vi "Cambridge Laser Control.vi"(7 "Calling VI Ref":refnum<vi>) -> ()   [LabVIEW 2016]
uses:
  Laser Controls/Laser Control.ctl
  Laser Controls/AOTF Control.ctl
  <vilib>/Utility/miscctls.llb/LVPointTypeDef.ctl
  Hardware Configuration/Hardware Configuration Controls/Device Type.ctl
  Hardware Configuration/Hardware Configuration Controls/Device Function.ctl
  Device Library/Lasers/Laser Controls/Laser Actions.ctl
  Device Library/AOTF and AOM/AOTF Controls/AOTF Actions.ctl
panel:
  in  "642 AOTF":T1 {"Power (%)" max=100 step=1 scale=0.0..100.0; "Digital Power (%)" max=100 step=1}
  in  "560 AOTF":T1 {"Power (%)" max=100 step=1 scale=0.0..100.0; "Digital Power (%)" max=100 step=1}
  in  "546 AOTF":T1 {"Power (%)" max=100 step=1 scale=0.0..100.0; "Digital Power (%)" max=100 step=1}
  in  "488 AOTF":T1 {"Power (%)" max=100 step=1 scale=0.0..100.0; "Digital Power (%)" max=100 step=1}
  in  "405 AOTF":T1 {"Power (%)" max=100 step=1 scale=0.0..100.0; "Digital Power (%)" max=100 step=1}
  in  "Lasers On/Off":bool
  in  "Quit":bool
  in  "642":T2
  in  "560":T2
  in  "546":T2
  in  "488":T2
  in  "405":T2
  # "Laser Status"
  # "Laser Emission"
  # "Laser Power"
  # "Capture Active"
  # "Power (%)"
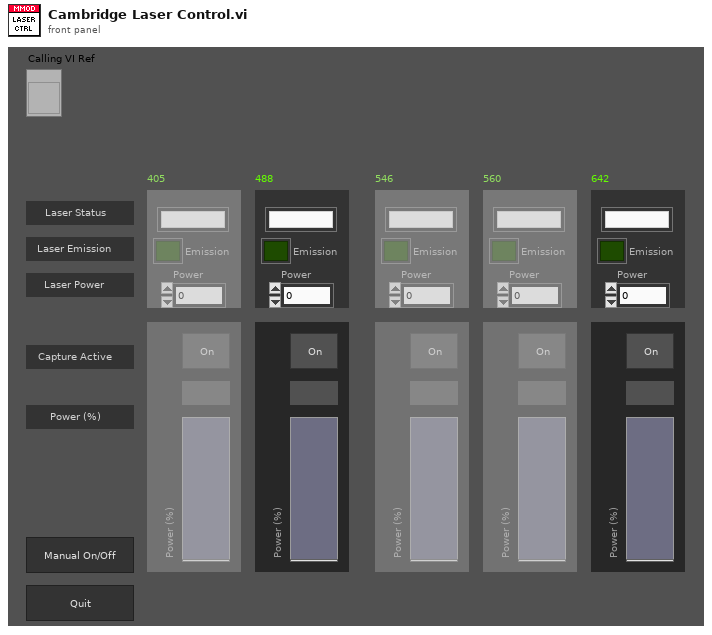
[diagram p1: front panel]
types:
  T1 = typedef "AOTF Control.ctl" = cluster{"Active":bool, "Digital Power (%)":u8, "Power (%)":u8}
  T2 = typedef "Laser Control.ctl" = cluster{"Status":string, "Emission":bool, "Power":dbl}
  T3 = enum16{"Always On", "Always Off", "Off While Running"}
  T4 = typedef "LVPointTypeDef.ctl" = cluster{"Horizontal":i16, "Vertical":i16}
  T5 = typedef "Device Function.ctl" = enum16{"Primary", "Secondary", "Overview", "Wide Field Drift Correction", "642 nm Excitation", "560 nm Excitation", "546 nm Excitation", "488 nm Excitation", "405 nm Excitation", "Objective Drift Correction", "Objective XY", "Objective Z", "Sample XY", "Sample Coarse Z", "Sample Z", "4Pi Lower", "4Pi Upper", "Adj Cavity"}
  T6 = typedef "Device Type.ctl" = enum16{"AOTF", "Camera", "Deformable Mirror", "Laser", "Shutter", "Stage"}
  T7 = typedef "Laser Actions.ctl" = enum16{"Error Check", "Set On/Off", "Set Power", "Set Parameter", "Get Power", "Get Status", "Get Parameter", "Quit"}
  T8 = enum8{"Enabled", "Disabled", "Disabled and Grayed Out"}
  T9 = typedef "AOTF Actions.ctl" = enum16{"Error Check", "Blank", "Line On/Off", "Set Power", "Status", "Quit"}
  T10 = typedef "Laser Status.ctl" = enum16{"Warmup", "Ready", "Emission", "Tuning", "Error"}
  T11 = cluster{"Status":bool, "Emission":bool, "Power":bool}
  T12 = cluster{"Active":bool, "Digital Power (%)":bool, "Power (%)":bool}
  T13 = typedef "LVRectTypeDef.ctl" = cluster{"Left":i16, "Top":i16, "Right":i16, "Bottom":i16}
  T14 = typedef "LVBoundsTypeDef.ctl" = cluster{"Width":u32, "Height":u32}
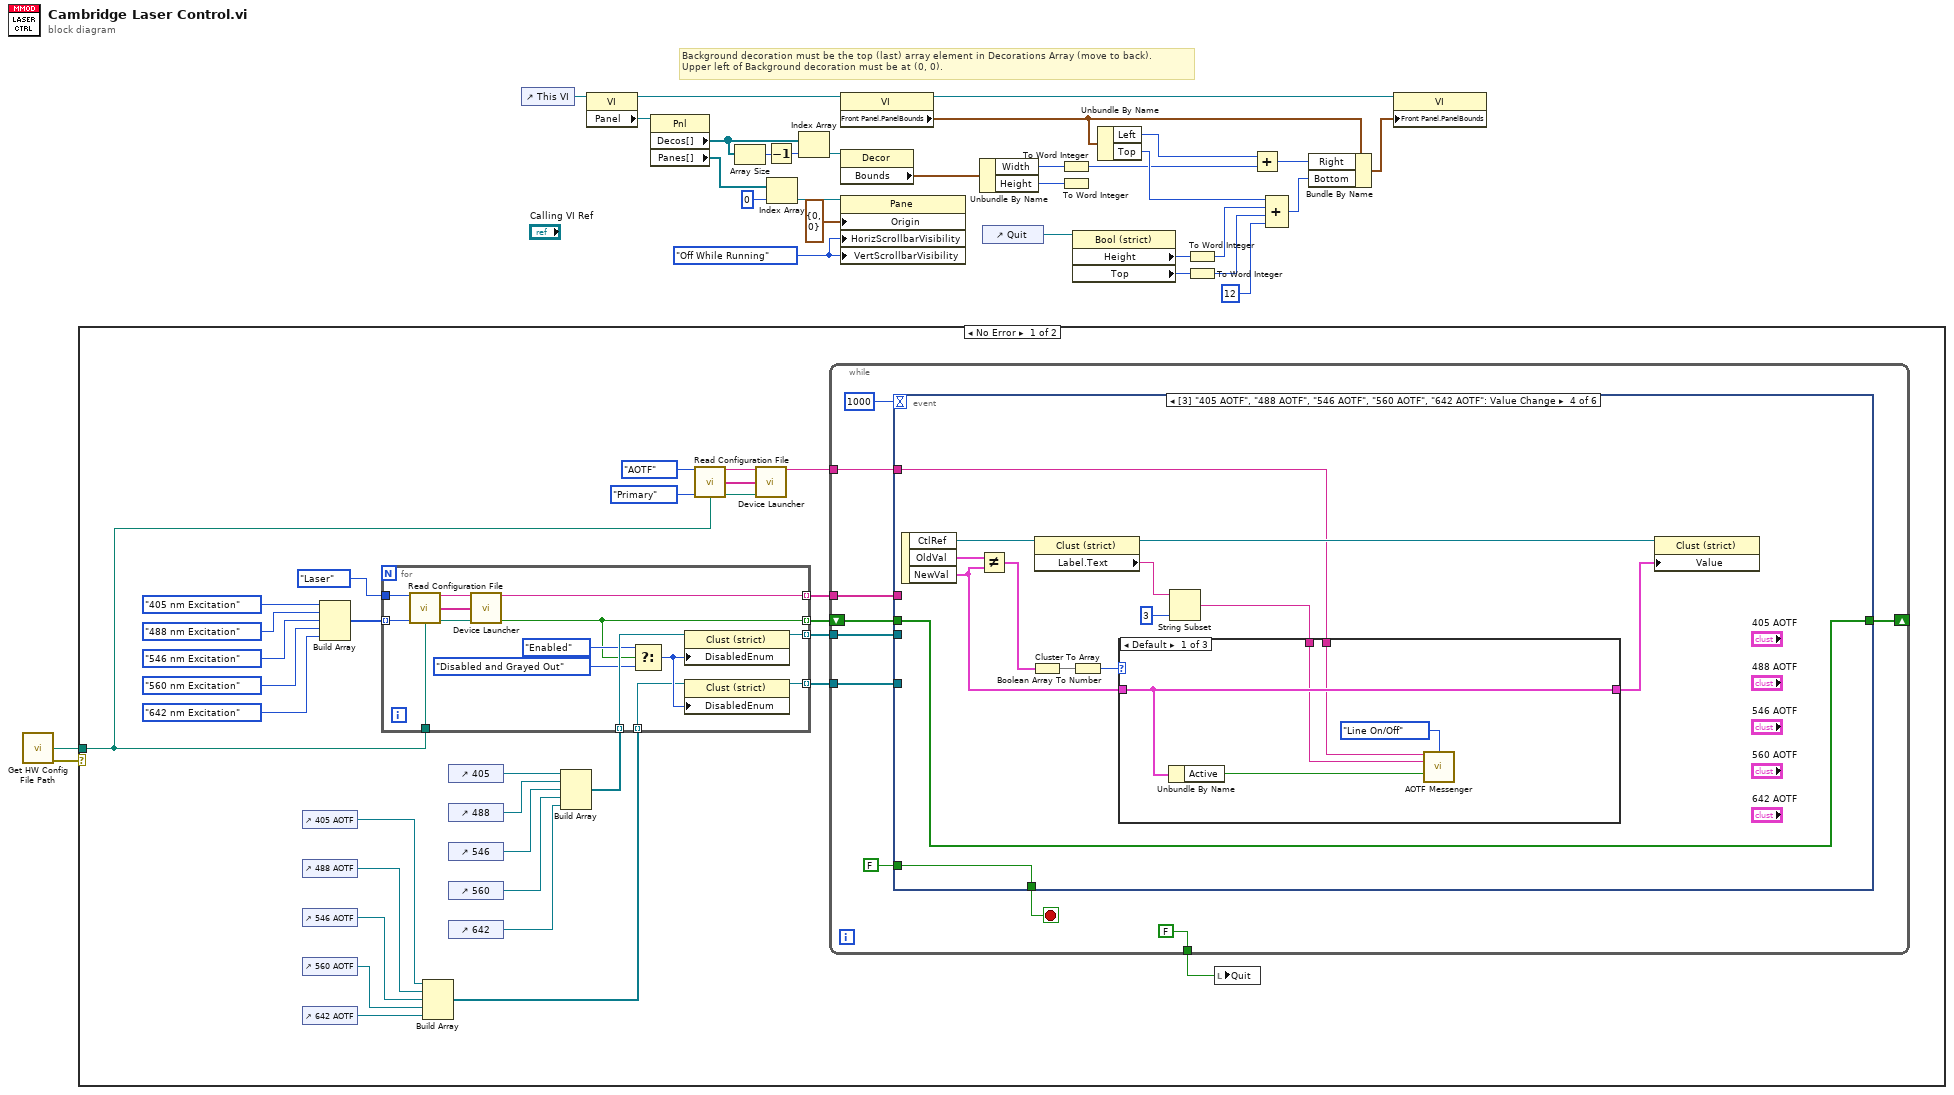
[diagram p0: block diagram]
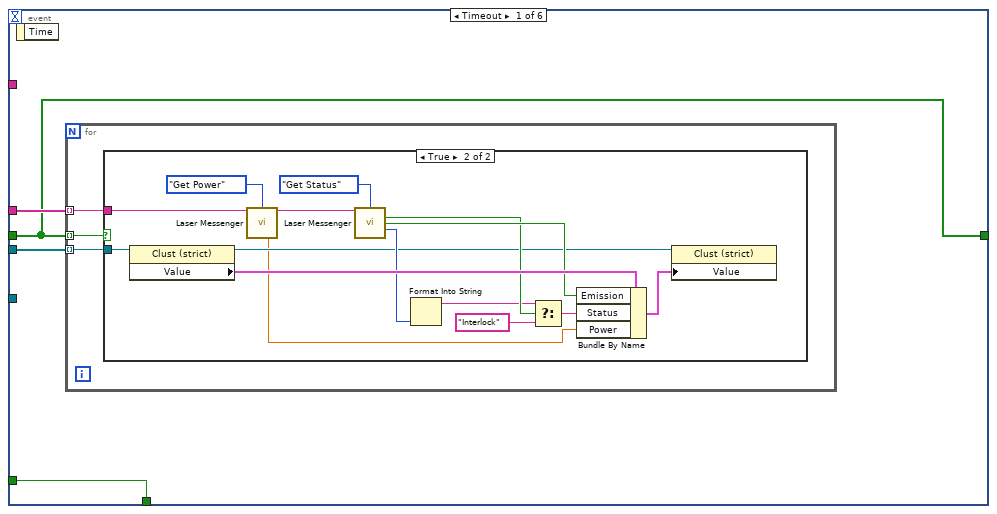
[diagram p2: hidden frame]
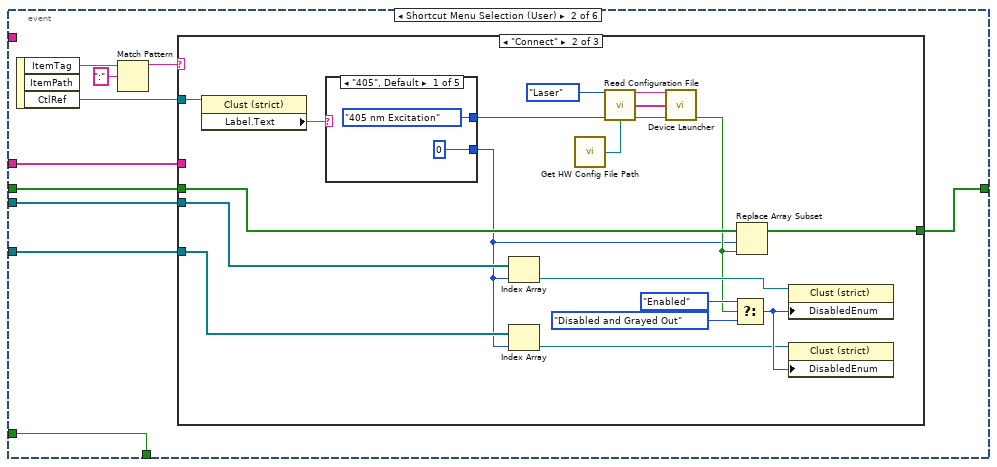
[diagram p4: hidden frame]
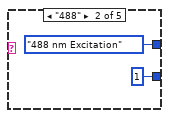
[diagram p6: hidden frame]
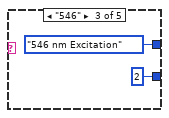
[diagram p7: hidden frame]
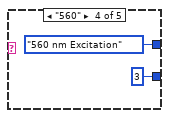
[diagram p8: hidden frame]
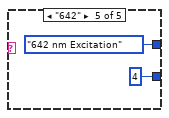
[diagram p9: hidden frame]
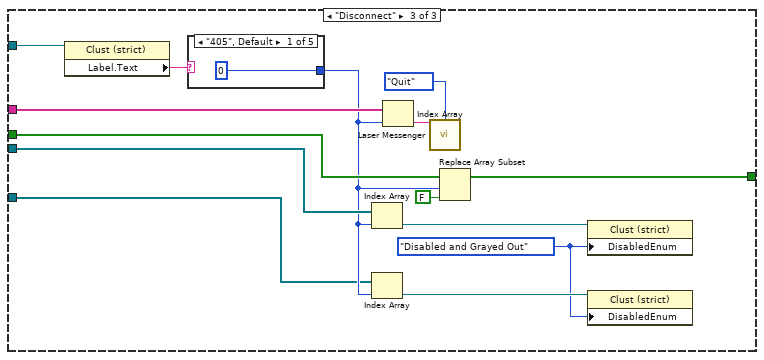
[diagram p10: hidden frame]
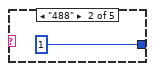
[diagram p11: hidden frame]
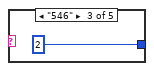
[diagram p12: hidden frame]
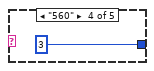
[diagram p13: hidden frame]
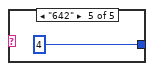
[diagram p14: hidden frame]
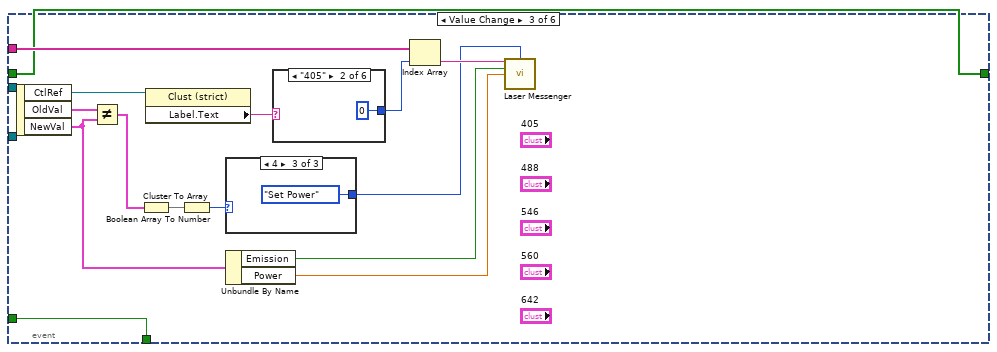
[diagram p15: hidden frame]
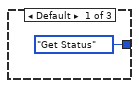
[diagram p16: hidden frame]
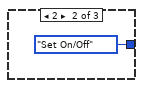
[diagram p17: hidden frame]
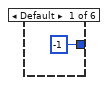
[diagram p18: hidden frame]
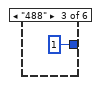
[diagram p19: hidden frame]
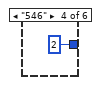
[diagram p20: hidden frame]
diagram:
  w12 = T3."Off While Running" ("Vertical Scrollbar Visibility")
  # "Background decoration must be the top (last) array element in Decorations Array (move to back).\nUpper left of Background decoration must be at (0, 0)."
  n1 = call "Get HW Config File Path.vi"() -> ("File Path"=w30:path, "Error"=w31:errorcluster)  [unwired: 14 in]
  n2 = case shown="No Error" w31 {
    tunnel: w30 -> [w32 _]
    frame No Error {
      n3 = control-ref of="405 AOTF"() -> (w42:refnum<vi>)
      n4 = control-ref of="488 AOTF"() -> (w43:refnum<vi>)
      n5 = control-ref of="546 AOTF"() -> (w44:refnum<vi>)
      n6 = control-ref of="560 AOTF"() -> (w45:refnum<vi>)
      n7 = control-ref of="642 AOTF"() -> (w46:refnum<vi>)
      n8 = Build Array(Device_Function."405 nm Excitation" ("Device Function"), Device_Function."488 nm Excitation" ("Device Function"), Device_Function."546 nm Excitation" ("Device Function"), Device_Function."560 nm Excitation" ("Device Function"), Device_Function."642 nm Excitation" ("Device Function")) -> (w56:T5[])
      n9 = Build Array(w42, w43, w44, w45, w46) -> (w41:refnum<vi>[])
      n10 = control-ref of="405"() -> (w51:refnum<vi>)
      n11 = control-ref of="488"() -> (w55:refnum<vi>)
      n12 = control-ref of="546"() -> (w54:refnum<vi>)
      n13 = control-ref of="560"() -> (w53:refnum<vi>)
      n14 = control-ref of="642"() -> (w52:refnum<vi>)
      n15 = Build Array(w51, w55, w54, w53, w52) -> (w50:refnum<vi>[])
      n16 = for {
        tunnel: [w236] -> w49 mode=indexing
        tunnel: Device_Type."Laser" ("Device Type") -> [w235]
        tunnel: w56 -> [w234] mode=indexing
        tunnel: w32 -> [w233]
        tunnel: w50 -> [w232] mode=indexing
        tunnel: [w229] -> w48 mode=indexing
        tunnel: [w228] -> w47 mode=indexing
        tunnel: w41 -> [w226] mode=indexing
        tunnel: [w225] -> w33 mode=indexing
        n17 = call "Read Configuration File.vi"("Device Type"=w235, "Device Function"=w234, "Config File Path"=w233) -> ("Unique Notifier Name"=w239:string, "Device Ports/IDs/Channels"=w237:string[], "Device Engine Path"=w238:path)  [unwired: 9 in, 1 out]
        n18 = call "Device Launcher.vi"("Notifier Name"=w239, "Device Ports/IDs/Channels"=w237, "Device Engine Path"=w238) -> ("Notifier Name"=w236:string, "Running?"=w229:bool)  [unwired: 11 in]
        n19 = Select(t=T8."Enabled" ("Disabled"), s=w229, f=T8."Disabled and Grayed Out") -> (s? t:f=w227:T8)
        n20 = property class="Clust (strict)"(reference=w232, "DisabledEnum"=w227) -> (reference out=w228:refnum<vi>)  [unwired: 1 in, 1 out]
        n21 = property class="Clust (strict)"(reference=w226, "DisabledEnum"=w227) -> (reference out=w225:refnum<vi>)  [unwired: 1 in, 1 out]
      }
      n22 = call "Read Configuration File.vi"("Device Type"=Device_Type."AOTF", "Device Function"=Device_Function."Primary", "Config File Path"=w32) -> ("Unique Notifier Name"=w38:string, "Device Ports/IDs/Channels"=w40:string[], "Device Engine Path"=w39:path)  [unwired: 9 in, 1 out]
      n23 = call "Device Launcher.vi"("Notifier Name"=w38, "Device Ports/IDs/Channels"=w40, "Device Engine Path"=w39) -> ("Notifier Name"=w35:string)  [unwired: 11 in, 1 out]
      n24 = while {
        tunnel: w49 -> [w71]
        tunnel: w47 -> [w67]
        shift-right: [w66] -> _
        shift-left: w48 -> [w70]
        tunnel: w35 -> [w65]
        tunnel: [FALSE] -> w34
        tunnel: w33 -> [w63]
        stop <- w68 stop-if-true
        n25 = event shown="[3] \"405 AOTF\", \"488 AOTF\", \"546 AOTF\", \"560 AOTF\", \"642 AOTF\": Value Change" {
          selector: _ -> [_ _ _ _ _ _]
          dyn-events: _ -> [_ _ _ _ _ _]
          timeout: 1000 -> [_ _ _ _ _ _]
          tunnel: w71 -> [w75 w96 w165 _ _ w218]
          tunnel: w70 -> [w73 w100 w154 w180 w212 w217]
          tunnel: FALSE -> [w76 w98 w168 w191 w215 _]
          tunnel: [w76 w98 w168 w191 w215 w219] -> w68
          tunnel: w67 -> [w74 w97 _ _ _ _]
          tunnel: [w73 w99 w154 w180 w212 w216] -> w66
          tunnel: w65 -> [_ _ _ w178 w214 _]
          tunnel: w63 -> [_ w95 _ _ _ _]
          event Timeout {
            n26 = event-data() -> ()  [unwired: 1 in, 1 out]
            n27 = for {
              tunnel: w75 -> [w78] mode=indexing
              tunnel: w73 -> [w79] mode=indexing
              tunnel: w74 -> [w77] mode=indexing
              n28 = case shown="True" w79 {
                tunnel: w78 -> [_ w84]
                tunnel: w77 -> [_ w93]
                frame False {
                }
                frame True {
                  n29 = property class="Clust (strict)"(reference=w93) -> (reference out=w85:refnum<vi>, "Value"=w92:T2)  [unwired: 1 in, 1 out]
                  n30 = call "Laser Messenger.vi"("Notifier Name"=w84, "Action"=Laser_Actions."Get Power") -> ("Notifier Name Dup"=w83:string, "Power (mW)"=w81:dbl)  [unwired: 8 in, 4 out]
                  n31 = call "Laser Messenger.vi"("Notifier Name"=w83, "Action"=Laser_Actions."Get Status") -> ("Enabled (Interlock)?"=w89:bool, "Light Emission?"=w91:bool, "Laser Status"=w90:T10)  [unwired: 8 in, 3 out]
                  n32 = Format Into String(w90) -> (resulting string=w88:string)  [unwired: 3 in, 1 out]
                  n33 = Select(t=w88, s=w89, f="Interlock") -> (s? t:f=w86:string)
                  n34 = Bundle By Name(cluster=w92, "Emission"=w91, "Status"=w86, "Power"=w81) -> (w80:T2)
                  n35 = property class="Clust (strict)"(reference=w85, "Value"=w80) -> ()  [unwired: 1 in, 2 out]
                }
              }
            }
          }
          event Shortcut Menu Selection (User) {
            n36 = event-data() -> ("ItemTag"=w103:string, "CtlRef"=w101:refnum<vi>)  [unwired: 1 in, 1 out]
            n37 = Match Pattern(string=w103, regular expression=":") -> (before substring=w102:string)  [unwired: 1 in, 3 out]
            n38 = case shown="\"Connect\"" w102 {
              tunnel: w101 -> [_ w124 w145]
              tunnel: w100 -> [w105 w117 w144]
              tunnel: [w105 w113 w142] -> w99
              tunnel: w97 -> [_ w112 w146]
              tunnel: w96 -> [_ _ w143]
              tunnel: w95 -> [_ w108 w137]
              frame Default {
              }
              frame "Connect" {
                n39 = property class="Clust (strict)"(reference=w124) -> ("Label.Text"=w123:string)  [unwired: 1 in, 2 out]
                n40 = case shown="\"405\", Default" w123 {
                  tunnel: [Device_Function."405 nm Excitation" ("Device Function") Device_Function."488 nm Excitation" ("Device Function") Device_Function."546 nm Excitation" ("Device Function") Device_Function."560 nm Excitation" ("Device Function") Device_Function."642 nm Excitation" ("Device Function")] -> w119
                  tunnel: [0 1 2 3 4] -> w107
                  frame "405", Default {
                  }
                  frame "488" {
                  }
                  frame "546" {
                  }
                  frame "560" {
                  }
                  frame "642" {
                  }
                }
                n41 = Index Array(array=w112, index=w107) -> (element=w111:refnum<vi>)
                n42 = Index Array(array=w108, index=w107) -> (element=w106:refnum<vi>)
                n43 = call "Get HW Config File Path.vi"() -> ("File Path"=w118:path)  [unwired: 14 in, 1 out]
                n44 = call "Read Configuration File.vi"("Device Type"=Device_Type."Laser", "Device Function"=w119, "Config File Path"=w118) -> ("Unique Notifier Name"=w120:string, "Device Ports/IDs/Channels"=w122:string[], "Device Engine Path"=w121:path)  [unwired: 9 in, 1 out]
                n45 = call "Device Launcher.vi"("Notifier Name"=w120, "Device Ports/IDs/Channels"=w122, "Device Engine Path"=w121) -> ("Running?"=w110:bool)  [unwired: 11 in, 1 out]
                n46 = Select(t=T8."Enabled" ("Disabled"), s=w110, f=T8."Disabled and Grayed Out") -> (s? t:f=w109:T8)
                n47 = Replace Array Subset(array=w117, new element=w110, index=w107) -> (w113:bool[])
                n48 = property class="Clust (strict)"(reference=w111, "DisabledEnum"=w109) -> ()  [unwired: 1 in, 2 out]
                n49 = property class="Clust (strict)"(reference=w106, "DisabledEnum"=w109) -> ()  [unwired: 1 in, 2 out]
              }
              frame "Disconnect" {
                w135 = T8."Disabled and Grayed Out" ("Disabled")
                n50 = property class="Clust (strict)"(reference=w145) -> ("Label.Text"=w148:string)  [unwired: 1 in, 2 out]
                n51 = case shown="\"405\", Default" w148 {
                  tunnel: [0 1 2 3 4] -> w138
                  frame "405", Default {
                  }
                  frame "488" {
                  }
                  frame "546" {
                  }
                  frame "560" {
                  }
                  frame "642" {
                  }
                }
                n52 = Index Array(array=w146, index=w138) -> (element=w147:refnum<vi>)
                n53 = Index Array(array=w137, index=w138) -> (element=w136:refnum<vi>)
                n54 = Index Array(array=w143, index=w138) -> (element=w141:string)
                n55 = call "Laser Messenger.vi"("Notifier Name"=w141, "Action"=Laser_Actions."Quit") -> ()  [unwired: 8 in, 6 out]
                n56 = Replace Array Subset(array=w144, new element=FALSE ("new element/subarray"), index=w138) -> (w142:bool[])
                n57 = property class="Clust (strict)"(reference=w147, "DisabledEnum"=w135) -> ()  [unwired: 1 in, 2 out]
                n58 = property class="Clust (strict)"(reference=w136, "DisabledEnum"=w135) -> ()  [unwired: 1 in, 2 out]
              }
            }
          }
          event Value Change {
            n59 = event-data() -> ("CtlRef"=w167:refnum<vi>, "OldVal"=w163:T2, "NewVal"=w157:T2)  [unwired: 1 in]
            n60 = Not Equal?(x=w163, y=w157) -> (x != y?=w158:T11)
            n61 = Cluster To Array(cluster=w158) -> (array=w162:bool[])
            n62 = property class="Clust (strict)"(reference=w167) -> ("Label.Text"=w166:string)  [unwired: 1 in, 2 out]
            n63 = Boolean Array To Number(Boolean array=w162) -> (number=w161:u32)
            n64 = case shown="4" w161 {
              tunnel: [Laser_Actions."Get Status" ("Action") Laser_Actions."Set On/Off" ("Action") Laser_Actions."Set Power" ("Action")] -> w159
              frame Default {
              }
              frame 2 {
              }
              frame 4 {
              }
            }
            n65 = Unbundle By Name(w157) -> ("Emission"=w155:bool, "Power"=w156:dbl)
            n66 = case shown="\"405\"" w166 {
              tunnel: [-1 0 1 2 3 4] -> w164
              frame Default {
              }
              frame "405" {
              }
              frame "488" {
              }
              frame "546" {
              }
              frame "560" {
              }
              frame "642" {
              }
            }
            n67 = Index Array(array=w165, index=w164) -> (element=w160:string)
            n68 = call "Laser Messenger.vi"("Notifier Name"=w160, "Action"=w159, "Emission On/Off"=w155, "Power (mW)"=w156) -> ()  [unwired: 6 in, 6 out]
          }
          event Value Change {
            n69 = event-data() -> ("CtlRef"=w188:refnum<vi>, "OldVal"=w187:T1, "NewVal"=w183:T1)  [unwired: 1 in]
            n70 = Not Equal?(x=w187, y=w183) -> (x != y?=w189:T12)
            n71 = Cluster To Array(cluster=w189) -> (array=w190:bool[])
            n72 = property class="Clust (strict)"(reference=w188) -> (reference out=w182:refnum<vi>, "Label.Text"=w186:string)  [unwired: 1 in, 1 out]
            n73 = Boolean Array To Number(Boolean array=w190) -> (number=w184:u32)
            n74 = String Subset(string=w186, length (rest)=3 ("length (rest)")) -> (substring=w179:string)  [unwired: 1 in]
            n75 = case shown="Default" w184 {
              tunnel: w183 -> [w196 w202 w210]
              tunnel: [w196 w203 w209] -> w181
              tunnel: w179 -> [w192 w200 w206]
              tunnel: w178 -> [w193 w199 w207]
              frame Default {
                n76 = Unbundle By Name(w196) -> ("Active"=w194:bool)
                n77 = call "AOTF Messenger.vi"("AOTF Notifier Name"=w193, "AOTF Action"=AOTF_Actions."Line On/Off", "Wavelength (nm)"=w192, "Line On/Off"=w194) -> ()  [unwired: 7 in, 5 out]
              }
              frame 2 {
                n78 = Unbundle By Name(w202) -> ("Digital Power (%)"=w198:u8)
                n79 = To Double Precision Float(number=w198) -> (double precision float=w197:dbl)
                n80 = Bundle By Name(cluster=w202, "Power (%)"=w198) -> (w203:T1)
                n81 = call "AOTF Messenger.vi"("AOTF Notifier Name"=w199, "AOTF Action"=AOTF_Actions."Set Power", "Wavelength (nm)"=w200, "Power (%)"=w197) -> ()  [unwired: 7 in, 5 out]
              }
              frame 4 {
                n82 = Unbundle By Name(w210) -> ("Power (%)"=w205:u8)
                n83 = To Double Precision Float(number=w205) -> (double precision float=w204:dbl)
                n84 = Bundle By Name(cluster=w210, "Digital Power (%)"=w205) -> (w209:T1)
                n85 = call "AOTF Messenger.vi"("AOTF Notifier Name"=w207, "AOTF Action"=AOTF_Actions."Set Power", "Wavelength (nm)"=w206, "Power (%)"=w204) -> ()  [unwired: 7 in, 5 out]
              }
            }
            n86 = property class="Clust (strict)"(reference=w182, "Value"=w181) -> ()  [unwired: 1 in, 2 out]
          }
          event "Lasers On/Off": Value Change {
            n87 = event-data() -> ()  [unwired: 1 in, 6 out]
            n88 = call "AOTF Messenger.vi"("AOTF Notifier Name"=w214, "AOTF Action"=AOTF_Actions."Blank", "Beam Blank"="Lasers On/Off") -> ()  [unwired: 8 in, 5 out]
          }
          event "Quit": Value Change {
            n89 = event-data() -> ("NewVal"=w219:bool)  [unwired: 1 in]
            n90 = for {
              tunnel: w218 -> [w221] mode=indexing
              tunnel: w217 -> [w220] mode=indexing
              tunnel: [w220] -> w216 mode=indexing
              n91 = case shown="True" w220 {
                tunnel: w221 -> [_ w224]
                frame False {
                }
                frame True {
                  n92 = call "Laser Messenger.vi"("Notifier Name"=w224, "Action"=Laser_Actions."Set On/Off", "Emission On/Off"=FALSE) -> ()  [unwired: 7 in, 6 out]
                }
              }
            }
          }
        }
      }
      n93 = local write "Quit"(w34) -> ()
    }
    frame Error {
    }
  }
  n94 = control-ref of="This VI"() -> (w4:refnum<vi>)
  n95 = property class="VI"(reference=w4) -> (reference out=w13:refnum<vi>, "Panel"=w5:refnum<vi>)  [unwired: 1 in, 1 out]
  n96 = property class="Pnl"(reference=w5) -> ("Decos[]"=w3:refnum<vi>[], "Panes[]"=w9:refnum<vi>[])  [unwired: 1 in, 2 out]
  n97 = Array Size(array=w3) -> (size(s)=w1:i32)
  n98 = Decrement(x=w1) -> (x-1=w2:i32)
  n99 = Index Array(array=w9, index=0) -> (element=w8:refnum<vi>)
  n100 = Index Array(array=w3, index=w2) -> (element=w11:refnum<vi>)
  n101 = property class="VI"(reference=w13) -> (reference out=w15:refnum<vi>, "Front Panel.PanelBounds"=w16:T13)  [unwired: 1 in, 1 out]
  n102 = property class="Decor"(reference=w11) -> ("Bounds"=w14:T14)  [unwired: 1 in, 2 out]
  n103 = property class="Pane"(reference=w8, "Origin"=T4 {"Horizontal"=0, "Vertical"=0}, "HorizScrollbarVisibility"=w12, "VertScrollbarVisibility"=w12) -> ()  [unwired: 1 in, 2 out]
  n104 = Unbundle By Name(w14) -> ("Width"=w19:u32, "Height"=w22:u32)
  n105 = control-ref of="Quit"() -> (w6:refnum<vi>)
  n106 = To Word Integer(number=w19) -> (16bit integer=w21:i16)
  n107 = To Word Integer(number=w22) -> ()  [unwired: 1 out]
  n108 = property class="Bool (strict)"(reference=w6) -> ("Height"=w24:u32, "Top"=w25:i32)  [unwired: 1 in, 2 out]
  n109 = Unbundle By Name(w16) -> ("Left"=w18:i16, "Top"=w29:i16)
  n110 = To Word Integer(number=w24) -> (16bit integer=w27:i16)
  n111 = To Word Integer(number=w25) -> (16bit integer=w28:i16)
  n112 = Add(x=w18, y=w21) -> (x+y=w20:i16)
  n113 = Compound Arithmetic op=ADD(w29, w27, w28, i16 12 ("y")) -> (w23:i16)
  n114 = Bundle By Name(cluster=w16, "Right"=w20, "Bottom"=w23) -> (w17:T13)
  n115 = property class="VI"(reference=w15, "Front Panel.PanelBounds"=w17) -> ()  [unwired: 1 in, 2 out]
